vi "ReadState.lvclass.vi"(8 "error in (no error)":errorcluster, 11 "GumballMachine in":refnum<class "GumballMachine.lvclass">) -> (0 "error out":errorcluster, 2 "State.lvclass":refnum<class "State.lvclass">, 3 "GumballMachine out":refnum<class "GumballMachine.lvclass">)   [LabVIEW 2013, in "GumballMachine.lvclass"]
uses:
  GumballMachine.lvclass
  State.lvclass/State.lvclass
  GumballMachine.lvclass/GumballMachine.ctl
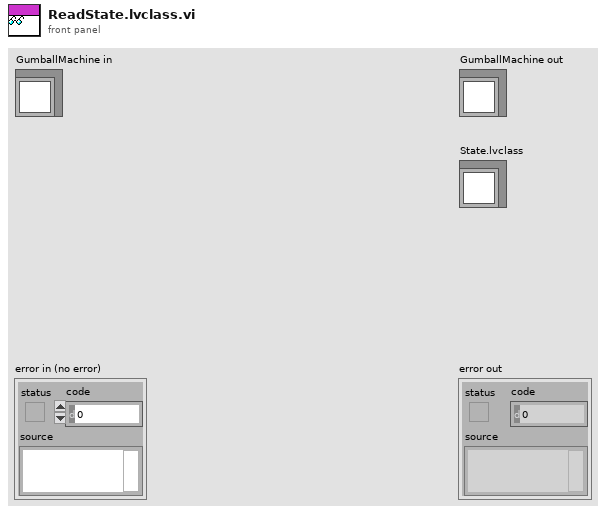
[diagram p1: front panel]
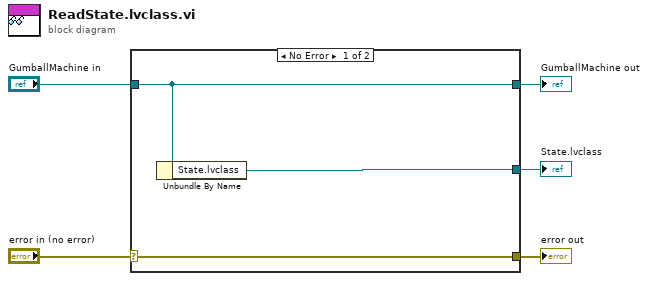
[diagram p0: block diagram]
diagram:
  n1 = case shown="No Error" "error in (no error)" {
    selector: "error in (no error)" -> [w8 w9]
    tunnel: [w8 w9] -> w4
    tunnel: [w7 w10] -> w2
    tunnel: "GumballMachine in" -> [w7 w10]
    tunnel: [w6 _] -> w1
    frame No Error {
      n2 = Unbundle By Name(w7) -> ("State.lvclass"=w6:refnum<class "State.lvclass">)
    }
    frame Error {
    }
  }
  "error out" <- w4
  "GumballMachine out" <- w2
  "State.lvclass" <- w1
